vi "DSF.Engine.Transceiver Thread.Main.vi"(8 "error in (no error)":errorcluster, 11 "Transceiver Thread in":refnum<class "DSF.Engine.Transceiver Thread.lvclass">) -> (0 "error out":errorcluster, 3 "Transceiver Thread out":refnum<class "DSF.Engine.Transceiver Thread.lvclass">)   [LabVIEW 2017, in "Data Sharing Framework Engine.lvlib" / "DSF.Engine.Transceiver Thread.lvclass"]
uses:
  DSF.Engine.Transceiver Thread.lvclass
  DSF.Engine.Transceiver Thread.lvclass/DSF.Engine.Transceiver Thread.ctl
  Thread Parameters/Thread Parameters.lvclass/Thread Parameters.ctl
  <vilib>/Platform/TimedLoop/XDataNode/timing_clust.ctl
  <vilib>/Platform/TimedLoop/XDataNode/nitl_modes.ctl
  <vilib>/Platform/TimedLoop/XDataNode/wakeup.ctl
  Interface/DSF.Engine.Interface.lvclass/DSF.Engine.Interface.ctl
  Source/Data Sharing Framework Core/Engine/Debug/Debug Flags FIFO/Debug Flags FIFO.lvclass/Debug Flags FIFO.ctl
  Transfer/DSF.Engine.Transfer Group.lvclass/DSF.Engine.Transfer Group.ctl
  Timing/DSF.Engine.Timing.lvclass/DSF.Engine.Timing.ctl
  Source/Data Sharing Framework Core/Engine/Debug/Debug Flags/Debug Flags.lvclass/Debug Flags.ctl
  Thread Pool/DSF.Engine.Pool.lvclass/DSF.Engine.Pool.ctl
  Transfer/DSF.Engine.Transfer.lvclass/DSF.Engine.Transfer.ctl
  Pointer/DSF.Engine.Pointer.DBL.lvclass/DSF.Engine.Pointer.DBL.ctl
  <vilib>/National Instruments/Memory Manager/Classes/Pointer/Memory.Pointer.lvclass/Memory.Pointer.ctl
  Interface/DSF.Engine.Interface.Transceiver.Read.vi
  Interface/DSF.Engine.Interface.Transceiver.Read.Command.vi
  DSF.Engine.Transceiver Thread.Get Interface.vi
  Transfer/DSF.Engine.Transfer Group.Return FIFO.Write.vi
  Thread Pool/DSF.Engine.Pool.ID.Return ID to Pool.vi
  DSF.Engine.Transceiver Thread.Get Thread ID Pool.vi
  Thread Parameters/Thread Parameters.Get ID.vi
  DSF.Engine.Transceiver.Command.Cast.Transfer Group.To.vi
  DSF.Engine.Transceiver Thread.Transfer Group.Get by ID.vi
  Transfer/DSF.Engine.Transfer Group.Set Current Iteration.vi
  Transfer/DSF.Engine.Transfer Group.Get Transfers.vi
  DSF.Engine.Transceiver Thread.Transfer.Build.vi
  Interface/DSF.Engine.Interface.Read.Command.vi
  Transfer/DSF.Engine.Transfer Group.Get Return FIFO.vi
  Transfer/DSF.Engine.Transfer Group.Get Timing.vi
  Timing/DSF.Engine.Timing.Get Iteration.vi
  Transfer/DSF.Engine.Transfer Group.Get Debug Flags.vi
  Source/Data Sharing Framework Core/Engine/Debug/Debug Flags/Get FIFO Flags.vi
  Source/Data Sharing Framework Core/Engine/Debug/Debug Flags FIFO/Get Infinite Timeouts.vi
  Thread Pool/DSF.Engine.Pool.Write FIFO.vi
  DSF.Engine.Transceiver Thread.Get Transfer Group.vi
  Timing/DSF.Engine.Timing.Iteration.Set.vi
  Transfer/DSF.Engine.Transfer Group.Set Timing.vi
  Buffer/DSF.Engine.Memory.Buffer.Insert Channels.Preserve Value.vi
  Transfer/DSF.Engine.Transfer.Get String Buffer.vi
  Transfer/DSF.Engine.Transfer.Get Intermediate Buffer.vi
  DSF.Engine.Transceiver Thread.Set Channels Buffer.vi
  DSF.Engine.Transceiver Thread.Get Channels Buffer.vi
  Transfer/DSF.Engine.Transfer.Get Channel Blocks.vi
  Pointer/DSF.Engine.Pointer.DBL.Read.vi
  Interface/DSF.Engine.Interface.Get Command FIFO.vi
  Interface/DSF.Engine.Interface.Get Debug Flags.vi
  Interface/DSF.Engine.Interface.RT FIFO.Read.16B.vi
  Thread Pool/DSF.Engine.Pool.Get FIFO.vi
  Thread Pool/DSF.Engine.Pool.Get Debug Flags.vi
  Timing/DSF.Engine.Timing.Set Iteration.vi
  Pointer/DSF.Engine.Pointer.DBL.Get Channel Count.vi
  <vilib>/National Instruments/Memory Manager/Classes/Pointer/Memory.Pointer.Read.vi
  <vilib>/National Instruments/Memory Manager/Classes/Pointer/Memory.Pointer.Read.1D.DBL.vi
  <vilib>/National Instruments/Memory Manager/Classes/Pointer/Memory.Pointer.Read.No Check.1D.DBL.vi
  <vilib>/National Instruments/Memory Manager/Classes/Pointer/Memory.Pointer.Parameter Check.Null Pointer.vi
  <vilib>/National Instruments/Memory Manager/Classes/Pointer/Memory.Pointer.Parameter Check.Subset.Power of 2.vi
  <vilib>/National Instruments/Memory Manager/Classes/Pointer/Memory.Pointer.Get Address.vi
  <vilib>/National Instruments/Memory Manager/Classes/Pointer/Memory.Pointer.Errors.vi
  <vilib>/National Instruments/Memory Manager/Classes/Pointer/Memory.Pointer.Errors.Null Pointer.vi
  <vilib>/National Instruments/Memory Manager/Classes/Pointer/Memory.Pointer.Errors.Out of Bounds.vi
  <vilib>/National Instruments/Memory Manager/Classes/Pointer/Memory.Pointer.Get Size.vi
  <vilib>/National Instruments/Memory Manager/Classes/Pointer/Memory.Pointer.Count to Size.Power of 2.vi
  <vilib>/National Instruments/Memory Manager/Classes/Pointer/Memory.Pointer.Errors.Create Error.vi
  <vilib>/NI/Static Error Handling/VIs/Static Error Handling.Source Buffer.Write.String.vi
  <vilib>/National Instruments/Memory Manager/Classes/Pointer/Memory.Pointer.Errors.Write Pointer Size.vi
  <vilib>/NI/Static Error Handling/VIs/Static Error Handling.Source Buffer.Write.Numeric.Scalar.Base10.vi
  <vilib>/NI/Static Error Handling/VIs/Static Error Handling.Source Buffer.Write.Numeric.Scalar.Base10 (U64).vi
  <vilib>/NI/Static Error Handling/VIs/Static Error Handling.Error Cluster Constant.vi
  <vilib>/NI/Static Error Handling/VIs/Static Error Handling.Error Cluster Constant (512B).vi
  <vilib>/NI/Static Error Handling/VIs/Static Error Handling.Parameters.Status.Set.vi
  <vilib>/NI/Static Error Handling/VIs/Static Error Handling.Parameters.Code.Set.vi
  <vilib>/NI/Static Error Handling/VIs/Static Error Handling.Parameters.VI Source.Set.vi
  <vilib>/National Instruments/Memory Manager/Constants/Memory.Constants.vi
  <vilib>/National Instruments/Memory Manager/Constants/Memory.Constants.Library Name.vi
  <vilib>/National Instruments/Memory Manager/Classes/Pointer/Memory.Pointer.Errors.Get Info.vi
  Interface/DSF.Engine.Interface.Transceiver.lvclass
  C:/github/data-sharing-framework/old/dsf core/Source/Engine/Classes/Interface/DSF.Engine.Interface.lvclass
  Thread Pool/DSF.Engine.Pool.ID.lvclass
  C:/github/data-sharing-framework/old/dsf core/Source/Engine/Classes/Thread Pool/DSF.Engine.Pool.lvclass
  Pointer/DSF.Engine.Pointer.DBL.lvclass
  C:/Program Files (x86)/National Instruments/LabVIEW 2017/vi.lib/National Instruments/Memory Manager/Classes/Pointer/Memory.Pointer.lvclass
  Buffer/DSF.Engine.Memory.Buffer.Write.vi
  Buffer/DSF.Engine.Memory.Buffer.Write.1D.U64.vi
  Buffer/DSF.Engine.Memory.Buffer.Write.1D.U32.vi
  Buffer/DSF.Engine.Memory.Buffer.Write.1D.U16.vi
  Buffer/DSF.Engine.Memory.Buffer.Write.1D.U8.vi
  Buffer/DSF.Engine.Memory.Buffer.Write.1D.I64.vi
  Buffer/DSF.Engine.Memory.Buffer.Write.1D.I32.vi
  Buffer/DSF.Engine.Memory.Buffer.Write.1D.I16.vi
  Buffer/DSF.Engine.Memory.Buffer.Write.1D.I8.vi
  Buffer/DSF.Engine.Memory.Buffer.Write.1D.DBL.vi
  Buffer/DSF.Engine.Memory.Buffer.Write.1D.SGL.vi
  Buffer/DSF.Engine.Memory.Buffer.Write.1D.Bool.vi
  <vilib>/platform/TimedLoop/XDataNode/XDataNode.xnode
  Thread Parameters/Thread Parameters.lvclass
  <vilib>/Platform/TimedLoop/XDataNode/XDNodeRunTimeDep.lvlib
panel:
  out "iteration":i32
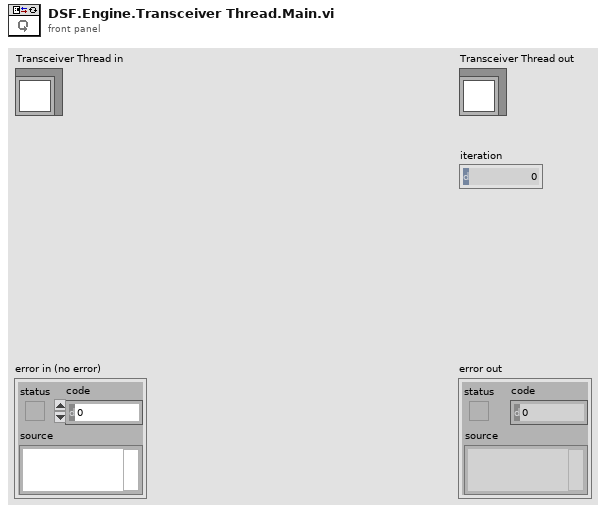
[diagram p1: front panel]
types:
  T1 = typedef "XDNodeRunTimeDep.lvlib/timing_clust.ctl" = cluster{"Expected End [f-1]":u64, "Actual End [f-1]":u64, "Finished Late? [f-1]":bool, "Expected End [i-1]":u64, "Actual End [i-1]":u64, "Finished Late? [i-1]":bool, "Expected Start [i]":u64, "Actual Start [i]":u64, "Expected Start [f]":u64, "Actual Start [f]":u64, "Source Name":string, "Structure Name":string, "Period":i64, "Deadline":i64, "Offset":i64, "Start":i64, "Priority":i32, "Timeout":i32, "Mode":T2, "Wakeup Reason":T3, "Error":errorcluster, "Source Type":string, "Secondary Source Type":string, "Global End Time":u64, "Global Start Time":u64, "Frame Duration":u64, "Iteration Duration":u64, "Assigned CPU":i32, "I/O Scan Engine Mode":u32}
  T2 = typedef "XDNodeRunTimeDep.lvlib/nitl_modes.ctl" = enum32{"No Change", "Process missed periods, maintain original phase", "Discard missed periods, maintain original phase", "Process missed periods, ignore original phase", "Discard missed periods, ignore original phase"}
  T3 = typedef "XDNodeRunTimeDep.lvlib/wakeup.ctl" = enum32{"Normal", "Aborted", "Asynchronous wakeup", "Timing source error", "Timed loop error", "Timeout"}
  T4 = typedef "Data Sharing Framework Engine.lvlib/DSF.Engine.Interface.Transceiver.lvclass/DSF.Engine.Interface.Transceiver.Command Data.ctl" = cluster{"Command":T5, "Command Parameters":T6}
  T5 = typedef "Data Sharing Framework Engine.lvlib/DSF.Engine.Interface.Transceiver.lvclass/DSF.Engine.Interface.Transceiver.Command.ctl" = enum8{"Set Base Pointer", "Rx", "Tx", "Shutdown"}
  T6 = typedef "Data Sharing Framework Engine.lvlib/DSF.Engine.Interface.Transceiver.lvclass/DSF.Engine.Interface.Transceiver.Command Parameters.ctl" = cluster{"arg1":u64, "arg2":u64}
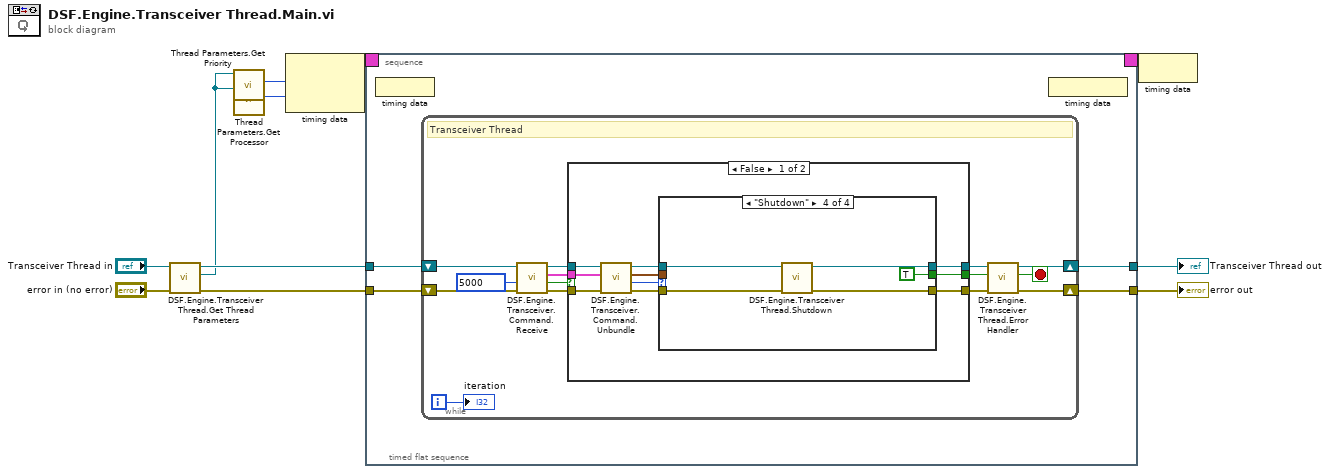
[diagram p0: block diagram]
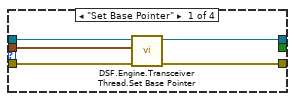
[diagram p2: hidden frame]
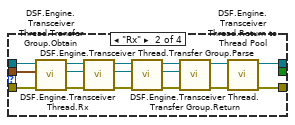
[diagram p3: hidden frame]
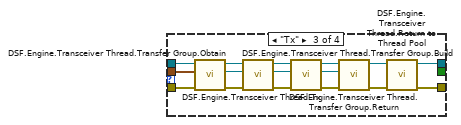
[diagram p4: hidden frame]
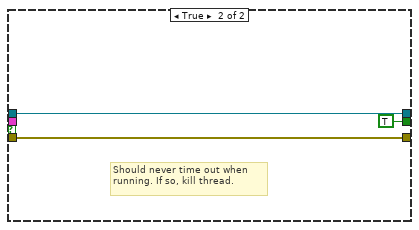
[diagram p5: hidden frame]
diagram:
  n1 = call "DSF.Engine.Transceiver Thread.Get Thread Parameters.vi"("Transceiver Thread in"="Transceiver Thread in") -> ("Thread Parameters"=w3:refnum<class "Thread Parameters.lvclass">, "Transceiver Thread out"=w4:refnum<class "DSF.Engine.Transceiver Thread.lvclass">)  [unwired: 9 in]
  n2 = call "Thread Parameters.Get Priority.vi"("Thread Parameters in"=w3) -> ("Priority"=w6:i32)  [unwired: 9 in, 1 out]
  n3 = call "Thread Parameters.Get Processor.vi"("Thread Parameters in"=w3) -> ("Processor"=w5:i32)  [unwired: 9 in, 1 out]
  n4 = node-c288(w6, w5) -> (w10:T1)
  n5 = timed-sequence {
    timing: w10 -> [_]
    timing-out: [_] -> w9
    tunnel: w4 -> [w14]
    tunnel: [w13] -> w8
    tunnel: "error in (no error)" -> [w12]
    tunnel: [w11] -> w1
    n6 = timed-flat-sequence {
      tunnel: w14 -> [w18]
      tunnel: [w17] -> w13
      tunnel: w12 -> [w16]
      tunnel: [w15] -> w11
      n7 = node-c288() -> ()  [unwired: 1 in]
      n8 = while {
        shift-right: [w22] -> w15
        shift-left: w16 -> [w30]
        shift-right: [w23] -> w17
        shift-left: w18 -> [w27]
        i -> [w19]
        stop <- w21 stop-if-true
        # "Transceiver Thread"
        n9 = call "DSF.Engine.Transceiver.Command.Receive.vi"("error in (no error)"=w30, "timeout in ms (0)"=5000 ("timeout in ms"), "Transceiver Thread in"=w27) -> ("error out"=w26:errorcluster, "timed out?"=w28:bool, "command"=w29:T4, "Transceiver Thread out"=w31:refnum<class "DSF.Engine.Transceiver Thread.lvclass">)  [unwired: 5 in]
        n10 = case shown="False" w28 {
          tunnel: w31 -> [w40 w87]
          tunnel: [w42 w87] -> w25
          tunnel: w26 -> [w39 w86]
          tunnel: w29 -> [w38 _]
          tunnel: [w41 w86] -> w24
          tunnel: [w33 TRUE] -> w20
          frame False {
            n11 = call "DSF.Engine.Transceiver.Command.Unbundle.vi"("error in (no error)"=w39, "command"=w38, "Transceiver Thread in"=w40) -> ("error out"=w36:errorcluster, "command"=w37:T5, "command parameters"=w34:T6, "Transceiver Thread out"=w35:refnum<class "DSF.Engine.Transceiver Thread.lvclass">)  [unwired: 5 in]
            n12 = case shown="\"Shutdown\"" w37 {
              tunnel: w35 -> [w47 w53 w69 w84]
              tunnel: [w46 w55 w72 w82] -> w42
              tunnel: w36 -> [w43 w48 w68 w83]
              tunnel: w34 -> [w44 w52 w65 _]
              tunnel: [w45 w54 w71 w81] -> w41
              tunnel: [_ _ _ TRUE] -> w33
              frame "Set Base Pointer" {
                n13 = call "DSF.Engine.Transceiver Thread.Set Base Pointer.vi"("error in (no error)"=w43, "command parameters"=w44, "Transceiver Thread in"=w47) -> ("error out"=w45:errorcluster, "Transceiver Thread out"=w46:refnum<class "DSF.Engine.Transceiver Thread.lvclass">)  [unwired: 7 in]
              }
              frame "Rx" {
                n14 = call "DSF.Engine.Transceiver Thread.Transfer Group.Obtain.vi"("error in (no error)"=w48, "command parameters"=w52, "Transceiver Thread in"=w53) -> ("error out"=w50:errorcluster, "Transfer Group"=w49:refnum<class "DSF.Engine.Transfer Group.lvclass">, "Transceiver Thread out"=w51:refnum<class "DSF.Engine.Transceiver Thread.lvclass">)  [unwired: 6 in]
                n15 = call "DSF.Engine.Transceiver Thread.Rx.vi"("error in (no error)"=w50, "Transfer Group in"=w49, "Transceiver Thread in"=w51) -> ("error out"=w62:errorcluster, "Transfer Group out"=w61:refnum<class "DSF.Engine.Transfer Group.lvclass">, "Transceiver Thread out"=w63:refnum<class "DSF.Engine.Transceiver Thread.lvclass">)  [unwired: 6 in]
                n16 = call "DSF.Engine.Transceiver Thread.Transfer Group.Parse.vi"("error in (no error)"=w62, "Transfer Group in"=w61, "Transceiver Thread in"=w63) -> ("error out"=w59:errorcluster, "Transfer Group out"=w58:refnum<class "DSF.Engine.Transfer Group.lvclass">, "Transceiver Thread out"=w60:refnum<class "DSF.Engine.Transceiver Thread.lvclass">)  [unwired: 6 in]
                n17 = call "DSF.Engine.Transceiver Thread.Transfer Group.Return.vi"("error in (no error)"=w59, "Transfer Group"=w58, "Transceiver Thread in"=w60) -> ("error out"=w56:errorcluster, "Transceiver Thread out"=w57:refnum<class "DSF.Engine.Transceiver Thread.lvclass">)  [unwired: 7 in]
                n18 = call "DSF.Engine.Transceiver Thread.Return to Thread Pool.vi"("error in (no error)"=w56, "Transceiver Thread in"=w57) -> ("error out"=w54:errorcluster, "Transceiver Thread out"=w55:refnum<class "DSF.Engine.Transceiver Thread.lvclass">)  [unwired: 8 in]
              }
              frame "Tx" {
                n19 = call "DSF.Engine.Transceiver Thread.Transfer Group.Obtain.vi"("error in (no error)"=w68, "command parameters"=w65, "Transceiver Thread in"=w69) -> ("error out"=w66:errorcluster, "Transfer Group"=w64:refnum<class "DSF.Engine.Transfer Group.lvclass">, "Transceiver Thread out"=w67:refnum<class "DSF.Engine.Transceiver Thread.lvclass">)  [unwired: 6 in]
                n20 = call "DSF.Engine.Transceiver Thread.Transfer Group.Build.vi"("error in (no error)"=w66, "Transfer Group in"=w64, "Transceiver Thread in"=w67) -> ("error out"=w78:errorcluster, "Transfer Group out"=w70:refnum<class "DSF.Engine.Transfer Group.lvclass">, "Transceiver Thread out"=w79:refnum<class "DSF.Engine.Transceiver Thread.lvclass">)  [unwired: 6 in]
                n21 = call "DSF.Engine.Transceiver Thread.Tx.vi"("error in (no error)"=w78, "Transfer Group in"=w70, "Transceiver Thread in"=w79) -> ("error out"=w76:errorcluster, "Transfer Group out"=w75:refnum<class "DSF.Engine.Transfer Group.lvclass">, "Transceiver Thread out"=w77:refnum<class "DSF.Engine.Transceiver Thread.lvclass">)  [unwired: 6 in]
                n22 = call "DSF.Engine.Transceiver Thread.Transfer Group.Return.vi"("error in (no error)"=w76, "Transfer Group"=w75, "Transceiver Thread in"=w77) -> ("error out"=w73:errorcluster, "Transceiver Thread out"=w74:refnum<class "DSF.Engine.Transceiver Thread.lvclass">)  [unwired: 7 in]
                n23 = call "DSF.Engine.Transceiver Thread.Return to Thread Pool.vi"("error in (no error)"=w73, "Transceiver Thread in"=w74) -> ("error out"=w71:errorcluster, "Transceiver Thread out"=w72:refnum<class "DSF.Engine.Transceiver Thread.lvclass">)  [unwired: 8 in]
              }
              frame "Shutdown" {
                n24 = call "DSF.Engine.Transceiver Thread.Shutdown.vi"("error in (no error)"=w83, "Transceiver Thread in"=w84) -> ("error out"=w81:errorcluster, "Transceiver Thread out"=w82:refnum<class "DSF.Engine.Transceiver Thread.lvclass">)  [unwired: 8 in]
              }
            }
          }
          frame True {
            # "Should never time out when running. If so, kill thread."
          }
        }
        n25 = call "DSF.Engine.Transceiver Thread.Error Handler.vi"("error in (no error)"=w24, "stop"=w20, "Transceiver Thread in"=w25) -> ("error out"=w22:errorcluster, "stop"=w21:bool, "Transceiver Thread out"=w23:refnum<class "DSF.Engine.Transceiver Thread.lvclass">)  [unwired: 6 in]
        "iteration" <- w19
      }
      n26 = node-c288() -> ()  [unwired: 1 out]
    }
  }
  "error out" <- w1
  "Transceiver Thread out" <- w8
  n27 = node-c288(w9) -> ()
